vi "Type Conversion.vi"(11 "Variant":variant) -> (3 "variant":variant)   [LabVIEW 2019, in "HDF5 Tools.lvlib"]
uses:
  HDF5 Tools.lvlib
  <vilib>/Utility/Data Type/NI_Data Type.lvlib
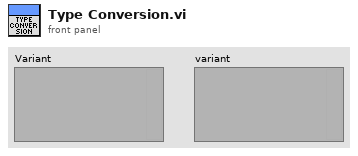
[diagram p1: front panel]
types:
  T1 = typedef "NI_Data Type.lvlib/Data Type.ctl" = enum8{"Invalid Type", "Void", "I8", "I16", "I32", "I64", "U8", "U16", "U32", "U64", "Single Float", "Double Float", "Extended Float", "Single Complex", "Double Complex", "Extended Complex", "Enum U8", "Enum U16", "Enum U32", "Enum U64", "Single Float With Unit", "Double Float With Unit", "Extended Float With Unit", "Single Complex with Unit", "Double Complex with Unit", "Extended Complex with Unit", "Boolean", "String", "Path", "Picture", "Tag", "Array", "Cluster", "Variant", "LV Variant", "Waveform", "Timestamp", "Digital Waveform", "Digital Data", "ExpressData", "Refnum", "External Data", "VI", "Poly VI", "LabVIEW Class Instance", "Fixed Point", "Set Collection", "Map Collection"}
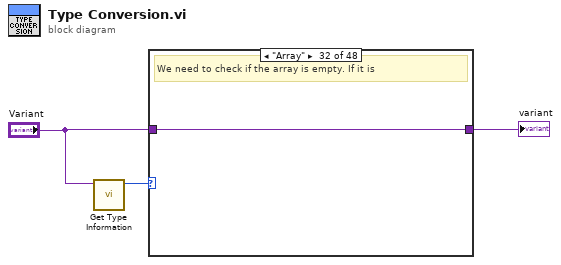
[diagram p0: block diagram]
diagram:
  n1 = call <vilib>:"Get Type Information.vi"("variant"="Variant") -> ("type"=w3:T1)  [unwired: 6 in, 4 out]
  n2 = case shown="\"Array\"" w3 {
    tunnel: "Variant" -> [w4 w5 w6 w7 w8 w9 w10 w11 w12 w13 w14 w15 w16 w17 w18 w19 w20 w21 w22 w23 w24 w25 w26 w27 w28 w29 w30 w31 w36 w37 w38 w39 w40 w41 w42 w43 w44 w45 w46 w47 w48 w49 w50 w51 w52 w53 w54 w55]
    tunnel: [w4 w5 w6 w7 w8 w9 w10 w11 w12 w13 w14 w15 w16 w17 w18 w19 w20 w21 w22 w23 w24 w25 w26 w27 w28 w29 w30 w31 w32 w37 w38 w39 w40 w41 w42 w43 w44 w45 w46 w47 w48 w49 w50 w51 w52 w53 w54 w55] -> w1
    frame "Invalid Type", Default {
    }
    frame "Void" {
    }
    frame "I8" {
    }
    frame "I16" {
    }
    frame "I32" {
    }
    frame "I64" {
    }
    frame "U8" {
    }
    frame "U16" {
    }
    frame "U32" {
    }
    frame "U64" {
    }
    frame "Single Float" {
    }
    frame "Double Float" {
    }
    frame "Extended Float" {
    }
    frame "Single Complex" {
    }
    frame "Double Complex" {
    }
    frame "Extended Complex" {
    }
    frame "Enum U8" {
    }
    frame "Enum U16" {
    }
    frame "Enum U32" {
    }
    frame "Enum U64" {
    }
    frame "Single Float With Unit" {
    }
    frame "Double Float With Unit" {
    }
    frame "Extended Float With Unit" {
    }
    frame "Single Complex with Unit" {
    }
    frame "Double Complex with Unit" {
    }
    frame "Extended Complex with Unit" {
    }
    frame "Boolean" {
    }
    frame "String" {
    }
    frame "Path" {
      n3 = Variant To Data(type=path "", Variant=w36) -> (data=w35:path)  [unwired: 1 in, 1 out]
      n4 = Path To String(path=w35) -> (string=w33:string)
      n5 = To Variant(anything=w33) -> (Variant=w32:variant)
    }
    frame "Picture" {
    }
    frame "Tag" {
    }
    frame "Array" {
      # "We need to check if the array is empty. If it is"
    }
    frame "Cluster" {
    }
    frame "Variant" {
    }
    frame "LV Variant" {
    }
    frame "Waveform" {
    }
    frame "Timestamp" {
    }
    frame "Digital Waveform" {
    }
    frame "Digital Data" {
    }
    frame "ExpressData" {
    }
    frame "Refnum" {
    }
    frame "External Data" {
    }
    frame "VI" {
    }
    frame "Poly VI" {
    }
    frame "LabVIEW Class Instance" {
    }
    frame "Fixed Point" {
    }
    frame "Set Collection" {
    }
    frame "Map Collection" {
    }
  }
  "variant" <- w1
